vi "Main UI.vi"() -> ()   [LabVIEW 2017]
uses:
  Type Defs/Tabs.ctl
  Type Defs/Saturation.ctl
  QSM/Expansion/Type Defs/Expansion.ctl
  Type Defs/Recipes.ctl
  QSM/Recipes/Type Defs/Recipes State.ctl
  QSM/Saturation/Type Defs/Saturation State.ctl
  QSM/Expansion/Type Defs/Expansion State.ctl
  QSM/Expansion/Expansion.lvclass
  QSM/Saturation/Saturation.lvclass
  QSM/Recipes/Recipes.lvclass
panel:
  in  "Hardware File Loaded":path
  in  "Configured Devices":T1(array[cluster])
  in  "Abort All":bool
  in  "Tabs":T2
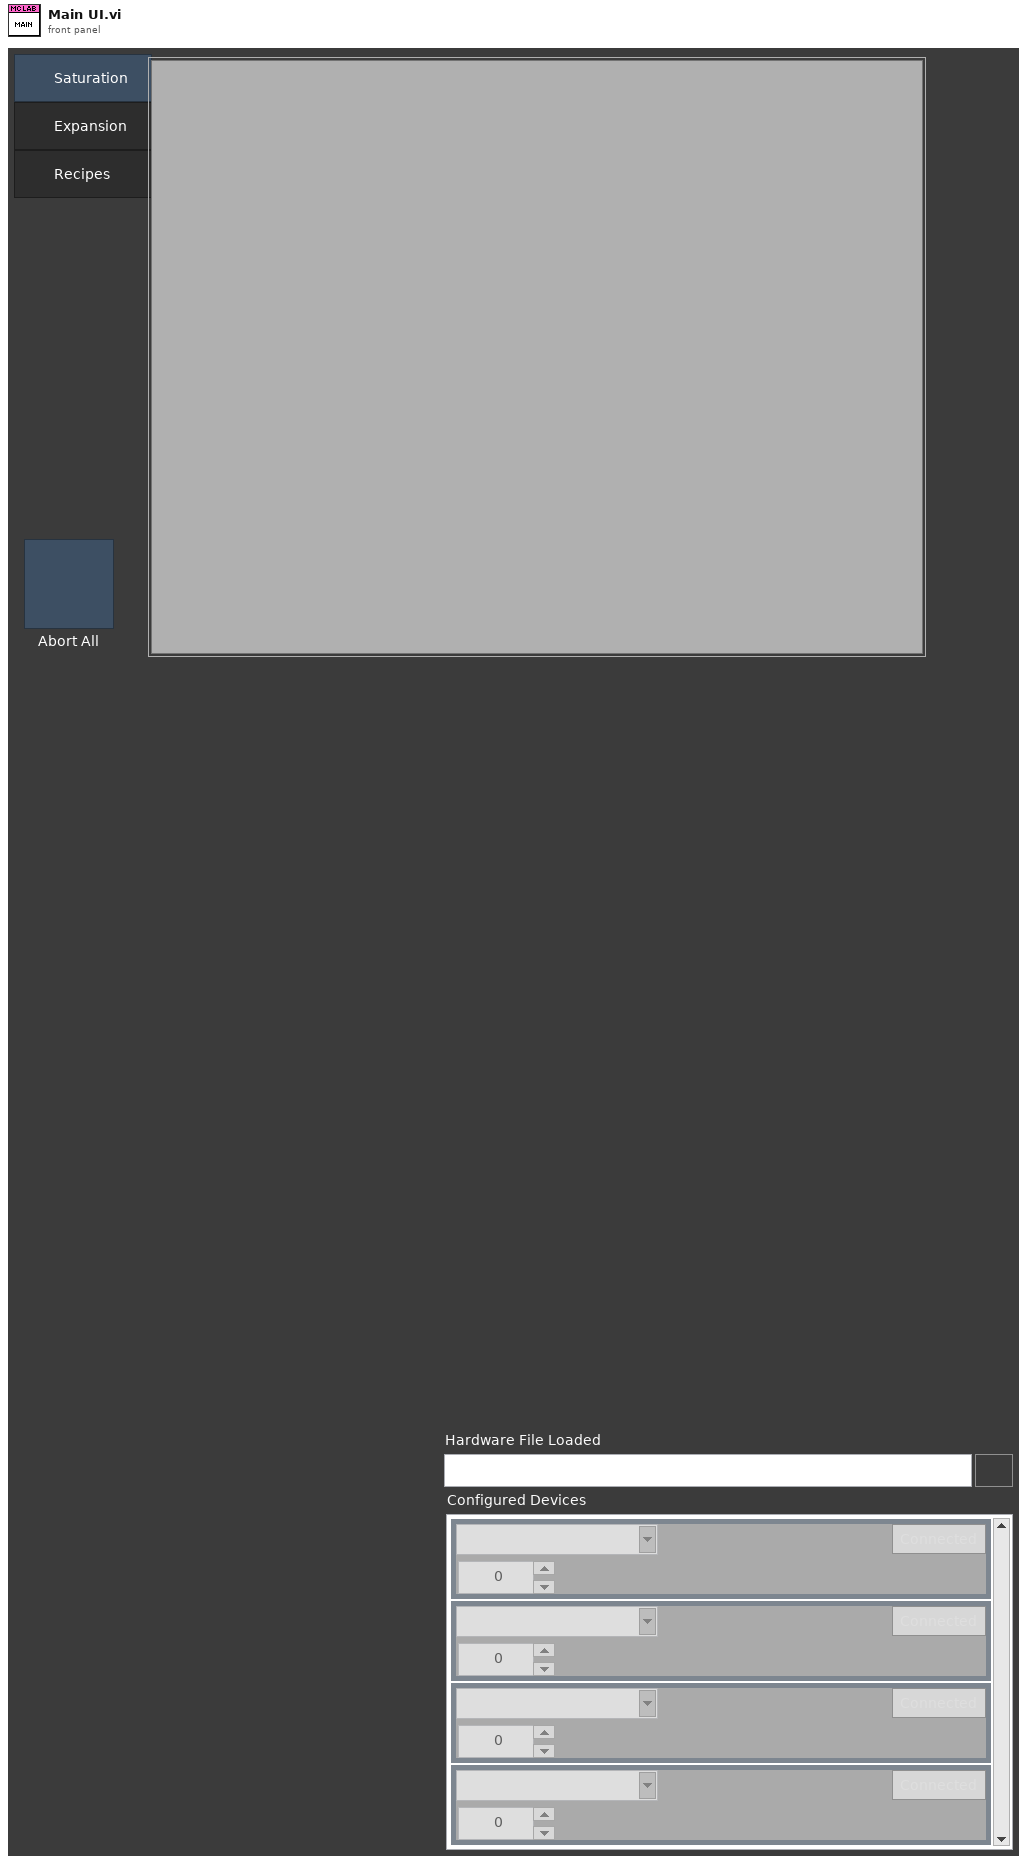
[diagram p1: front panel]
types:
  T1 = cluster{"DAQmx Task Name":refnum<k21>, "Sample Rate":dbl, "HW Connected":bool}[]
  T2 = typedef "Tabs.ctl" = enum32{"Saturation", "Expansion", "Recipes"}
  T3 = typedef "Recipes.lvclass/Recipes State.ctl" = enum16{"Init", "Update List", "Create", "Send", "Load", "Save", "Idle", "Error", "Shutdown"}
  T4 = typedef "Expansion.lvclass/Expansion State.ctl" = enum16{"Init", "Update", "Go", "Move from Load to Heating", "Stop Motor", "Operate Cylinders", "Wait and Monitor", "Move from Heating to Unload", "Unload", "Move from Unload to Heating", "Move from Heating to Load", "Complete Process", "Stop", "Idle", "Error", "Shutdown"}
  T5 = typedef "Saturation.lvclass/Saturation State.ctl" = enum16{"Init", "Update", "Go", "Control Valve", "Wait for Pressure", "Wait and Monitor", "Stop", "Idle", "Error", "Shutdown"}
  T6 = enum32{"Bad", "Idle", "Run top level", "Running"}
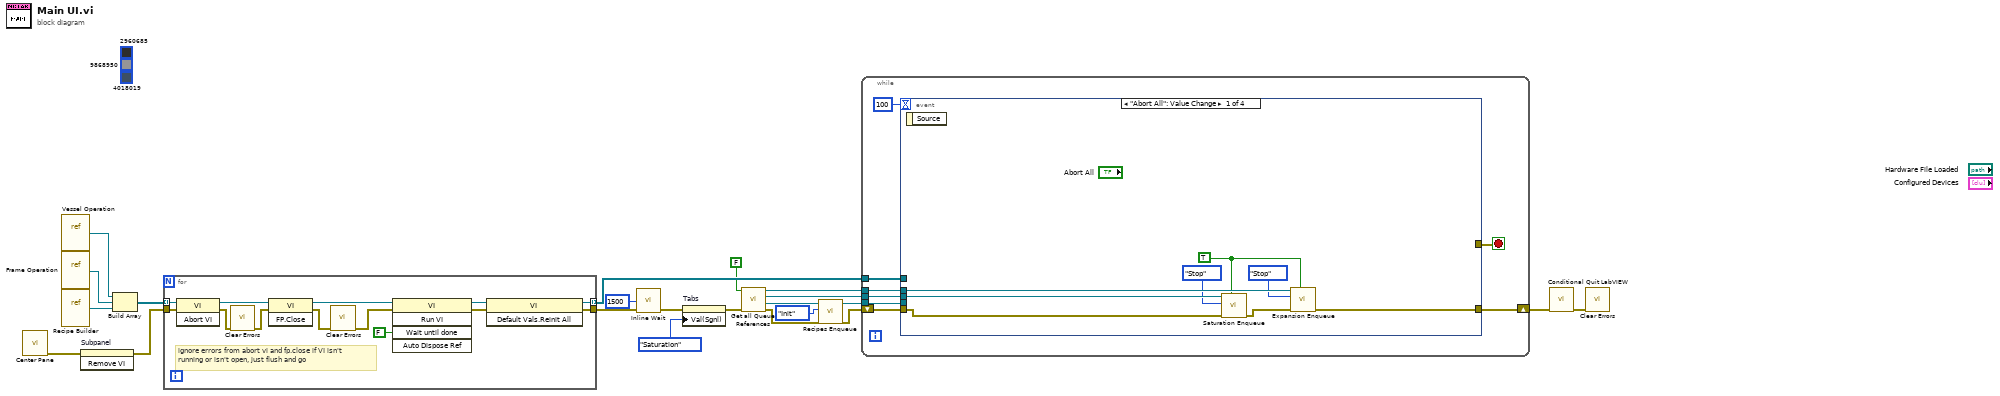
[diagram p0: block diagram]
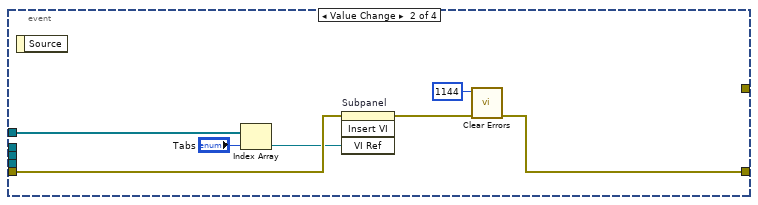
[diagram p2: hidden frame]
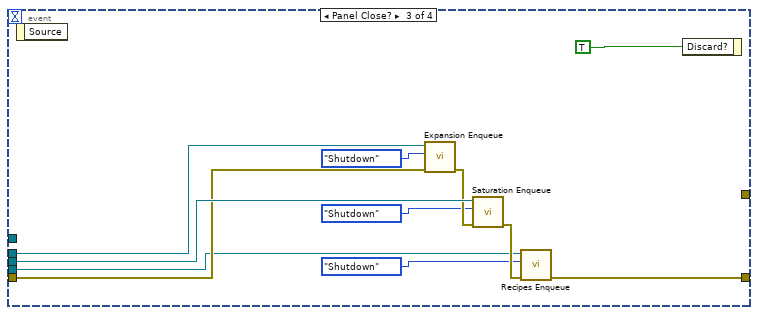
[diagram p3: hidden frame]
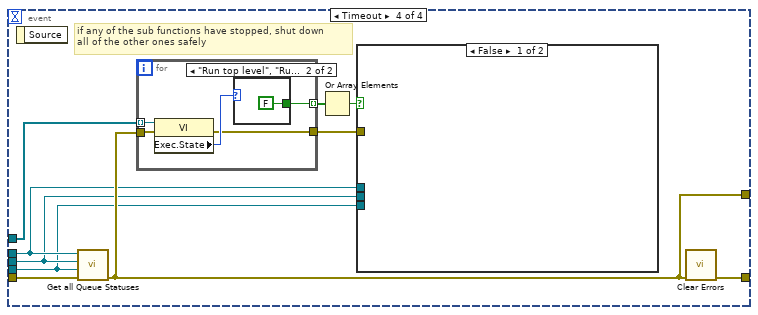
[diagram p4: hidden frame]
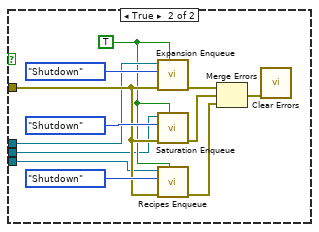
[diagram p5: hidden frame]
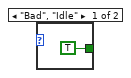
[diagram p6: hidden frame]
diagram:
  (unwired) u32 4018019 ("Color Box 2")
  (unwired) u32 9868950 ("Color Box 3")
  (unwired) u32 2960685 ("Color Box")
  n1 = call "Center Pane.vi"() -> ("error out"=w8:errorcluster)  [unwired: 11 in]
  n2 = vi-ref "Vessel Operation.vi"() -> (w12:refnum<vi>)
  n3 = vi-ref "Frame Operation.vi"() -> (w11:refnum<vi>)
  n4 = vi-ref "Recipe Builder.vi"() -> (w10:refnum<vi>)
  n5 = invoke on="Subpanel" class="SubPnl" method="Remove VI"(error in=w8) -> (error out=w16:errorcluster)  [unwired: 2 in, 2 out]
  n6 = Build Array(w12, w11, w10) -> (w19:refnum<vi>[])
  n7 = for {
    tunnel: w19 -> [w34] mode=indexing
    tunnel: [w25] -> w18 mode=indexing
    tunnel: w16 -> [w33]
    tunnel: [w23] -> w17
    # "ignore errors from abort vi and fp.close if VI isn't running or isn't open, just flush and go"
    n8 = invoke class="VI" method="Abort VI"(reference=w34, error in=w33) -> (reference out=w31:refnum<vi>, error out=w30:errorcluster)  [unwired: 1 in, 1 out]
    n9 = call <vilib>:"Clear Errors.vi"("error in (no error)"=w30) -> ("error out"=w27:errorcluster)  [unwired: 5 in, 1 out]
    n10 = invoke class="VI" method="FP.Close"(reference=w31, error in=w27) -> (reference out=w29:refnum<vi>, error out=w28:errorcluster)  [unwired: 1 in, 1 out]
    n11 = call <vilib>:"Clear Errors.vi"("error in (no error)"=w28) -> ("error out"=w32:errorcluster)  [unwired: 5 in, 1 out]
    n12 = invoke class="VI" method="Run VI"(reference=w29, error in=w32, "Wait until done"=FALSE ("Wait Until Done")) -> (reference out=w26:refnum<vi>, error out=w24:errorcluster)  [unwired: 2 in, 3 out]
    n13 = invoke class="VI" method="Default Vals.Reinit All"(reference=w26, error in=w24) -> (reference out=w25:refnum<vi>, error out=w23:errorcluster)  [unwired: 1 in, 1 out]
  }
  n14 = call "Inline Wait.vi"("error in (no error)"=w17, "Numeric"=u32 1500) -> ("error out"=w7:errorcluster)  [unwired: 3 in]
  n15 = property on="Tabs" class="RadioBtnsControl (strict)"(error in=w7, "Val(Sgnl)"=Tabs."Saturation" ("Tabs")) -> (error out=w9:errorcluster)  [unwired: 1 in, 1 out]
  n16 = call "Get all Queue References.vi"("error in (no error)"=w9, "create if not found? (F)"=FALSE ("create if not found? (T)")) -> ("error out"=w4:errorcluster, "Recipes Queue"=w5:refnum<queue>, "Saturation Queue"=w21:refnum<queue>, "Expansion Queue"=w22:refnum<queue>)  [unwired: 6 in]
  n17 = call "Recipes Enqueue.vi"("error in (no error)"=w4, "State"=Recipes_State."Init", "Queue in"=w5) -> ("error out"=w3:errorcluster, "Queue out"=w2:refnum<queue>)  [unwired: 7 in]
  n18 = while {
    tunnel: w22 -> [w41]
    shift-right: [w39] -> w14
    shift-left: w3 -> [w40]
    tunnel: w21 -> [w38]
    tunnel: w18 -> [w37]
    tunnel: w2 -> [w36]
    stop <- w43 stop-if-true
    n19 = event shown="[0] \"Abort All\": Value Change" {
      selector: _ -> [_ _ _ _]
      dyn-events: _ -> [_ _ _ _]
      timeout: 100 -> [_ _ _ _]
      tunnel: [_ _ _ w74] -> w43
      tunnel: w41 -> [w50 _ w69 w72]
      tunnel: w40 -> [w47 w58 w64 w78]
      tunnel: [w48 w55 w65 w79] -> w39
      tunnel: w38 -> [w51 _ w68 w71]
      tunnel: w37 -> [_ w56 _ w77]
      tunnel: w36 -> [_ _ w63 w70]
      event "Abort All": Value Change {
        w44 = TRUE ("Opposite End?")
        n20 = event-data() -> ()  [unwired: 1 in, 1 out]
        n21 = call "Saturation Enqueue.vi"("Opposite End?"=w44, "error in (no error)"=w47, "State"=Saturation_State."Stop", "Queue in"=w51) -> ("error out"=w49:errorcluster)  [unwired: 6 in, 1 out]
        n22 = call "Expansion Enqueue.vi"("Opposite End? (F)"=w44, "error in (no error)"=w49, "State"=Expansion_State."Stop", "Queue in"=w50) -> ("error out"=w48:errorcluster)  [unwired: 6 in, 1 out]
      }
      event Value Change {
        n23 = event-data() -> ()  [unwired: 1 in, 1 out]
        n24 = Index Array(array=w56, index="Tabs") -> (element=w52:refnum<vi>)
        n25 = invoke on="Subpanel" class="SubPnl" method="Insert VI"(error in=w58, "VI Ref"=w52) -> (error out=w57:errorcluster)  [unwired: 2 in, 3 out]
        n26 = call <vilib>:"Clear Errors.vi"("error in (no error)"=w57, "specific error code to clear (0: all)"=1144) -> ("error out"=w55:errorcluster)  [unwired: 4 in, 1 out]
      }
      event Panel Close? {
        n27 = event-data() -> ()  [unwired: 1 in, 1 out]
        n28 = call "Expansion Enqueue.vi"("error in (no error)"=w64, "State"=Expansion_State."Shutdown", "Queue in"=w69) -> ("error out"=w67:errorcluster)  [unwired: 7 in, 1 out]
        n29 = call "Saturation Enqueue.vi"("error in (no error)"=w67, "State"=Saturation_State."Shutdown", "Queue in"=w68) -> ("error out"=w66:errorcluster)  [unwired: 7 in, 1 out]
        n30 = call "Recipes Enqueue.vi"("error in (no error)"=w66, "State"=Recipes_State."Shutdown", "Queue in"=w63) -> ("error out"=w65:errorcluster)  [unwired: 7 in, 1 out]
        n31 = event-data("Discard?"=TRUE) -> ()  [unwired: 1 in, 1 out]
      }
      event Timeout {
        # "if any of the sub functions have stopped, shut down\nall of the other ones safely"
        n32 = event-data() -> ()  [unwired: 1 in, 1 out]
        n33 = call "Get all Queue Statuses.vi"("error in (no error)"=w78, "Recipes Queue"=w70, "Saturation Queue"=w71, "Expansion Queue"=w72) -> ("error out"=w74:errorcluster)  [unwired: 7 in]
        n34 = for {
          tunnel: w77 -> [w96] mode=indexing
          tunnel: [w94] -> w76 mode=indexing
          tunnel: w74 -> [w93]
          tunnel: [w92] -> w73
          n35 = property class="VI"(reference=w96, error in=w93) -> (error out=w92:errorcluster, "Exec.State"=w95:T6)  [unwired: 1 out]
          n36 = case shown="\"Run top level\", \"Running\"" w95 {
            tunnel: [TRUE FALSE] -> w94
            frame "Bad", "Idle" {
            }
            frame "Run top level", "Running" {
            }
          }
        }
        n37 = Or Array Elements(Boolean array=w76) -> (logical OR=w75:bool)
        n38 = case shown="False" w75 {
          tunnel: w73 -> [_ w86]
          tunnel: w72 -> [_ w85]
          tunnel: w71 -> [_ w81]
          tunnel: w70 -> [_ w80]
          frame False {
          }
          frame True {
            w82 = TRUE ("Opposite End?")
            n39 = call "Expansion Enqueue.vi"("Opposite End? (F)"=w82, "error in (no error)"=w86, "State"=Expansion_State."Shutdown", "Queue in"=w85) -> ("error out"=w84:errorcluster)  [unwired: 6 in, 1 out]
            n40 = call "Saturation Enqueue.vi"("Opposite End?"=w82, "error in (no error)"=w86, "State"=Saturation_State."Shutdown", "Queue in"=w81) -> ("error out"=w83:errorcluster)  [unwired: 6 in, 1 out]
            n41 = call "Recipes Enqueue.vi"("Opposite End?"=w82, "error in (no error)"=w86, "State"=Recipes_State."Shutdown", "Queue in"=w80) -> ("error out"=w87:errorcluster)  [unwired: 6 in, 1 out]
            n42 = Merge Errors(w84, w83, w87) -> (w88:errorcluster)
            n43 = call <vilib>:"Clear Errors.vi"("error in (no error)"=w88) -> ()  [unwired: 5 in, 2 out]
          }
        }
        n44 = call <vilib>:"Clear Errors.vi"("error in (no error)"=w74) -> ("error out"=w79:errorcluster)  [unwired: 5 in, 1 out]
      }
    }
  }
  n45 = call "Conditional Quit LabVIEW.vi"("error in (no error)"=w14) -> ("error out"=w13:errorcluster)  [unwired: 10 in]
  n46 = call <vilib>:"Clear Errors.vi"("error in (no error)"=w13) -> ()  [unwired: 5 in, 2 out]
